vi "Framework.Create.Transfers.vi"(5 "Group String Buffer":refnum<class "Buffer.lvclass">, 7 "Group Intermediate Buffer":refnum<class "DBL Pointer.lvclass">, 8 "error in (no error)":errorcluster, 10 "Transfer Configurations":refnum<class "Transfer Configuration.lvclass">[](array[class]), 11 "Framework in":refnum<class "Framework.lvclass">) -> (0 "error out":errorcluster, 2 "Transfers":refnum<class "Transfer.lvclass">[](array[class]), 3 "Framework out":refnum<class "Framework.lvclass">)   [LabVIEW 2017, in "DSF Core.lvlib" / "Framework.lvclass"]
uses:
  Framework.lvclass
  Transfer/Transfer.lvclass
  Shared/Classes/Transfer/Transfer Configuration.lvclass
  Buffer/Buffer.lvclass
  C:/Program Files (x86)/National Instruments/LabVIEW 2017/vi.lib/NI/Memory Manager/Classes/Pointer/Memory.Pointer.lvclass
  Pointer/DBL Pointer.lvclass
  Framework.lvclass/Framework.ctl
  Cache/Cache.lvclass/Cache.ctl
  DSF Configuration API/Public/Controls/DSF Data Type.ctl
  <vilib>/NI/Memory Manager/Classes/Pointer/Memory.Pointer.lvclass/Memory.Pointer.ctl
  Shared/Classes/Transfer/Transfer Configuration.lvclass/Transfer Configuration.ctl
  Shared/VIs/Data Type.Sizeof.vi
  <vilib>/NI/Memory Manager/Classes/Pointer/Memory.Pointer.Parameter Check.Subset.vi
  <vilib>/NI/Memory Manager/Classes/Pointer/Memory.Pointer.Get Address.vi
  <vilib>/NI/Memory Manager/Classes/Pointer/Memory.Pointer.Encapsulate.vi
  <vilib>/NI/Memory Manager/Classes/Pointer/Memory.Pointer.Parameter Check.Null Pointer.vi
  <vilib>/NI/Memory Manager/Classes/Pointer/Memory.Pointer.Errors.vi
  <vilib>/NI/Memory Manager/Classes/Pointer/Memory.Pointer.Errors.Out of Bounds.vi
  <vilib>/NI/Memory Manager/Classes/Pointer/Memory.Pointer.Get Size.vi
  <vilib>/NI/Memory Manager/Classes/Pointer/Memory.Pointer.Set Size.vi
  <vilib>/NI/Memory Manager/Classes/Pointer/Memory.Pointer.Set Address.vi
  <vilib>/NI/Memory Manager/Classes/Pointer/Memory.Pointer.Set Allocated.vi
  <vilib>/NI/Memory Manager/Classes/Pointer/Memory.Pointer.Errors.Null Pointer.vi
  <vilib>/NI/Memory Manager/VIs/Source.Write.String.vi
  <vilib>/NI/Memory Manager/Classes/Pointer/Memory.Pointer.Errors.Write Pointer Size.vi
  <vilib>/NI/Memory Manager/Classes/Pointer/Memory.Pointer.Errors.Create Error.vi
  <vilib>/NI/Memory Manager/VIs/Source.Write.Scalar.Base10.vi
  <vilib>/NI/Memory Manager/VIs/Source.Write.Scalar.Base10 (U64).vi
  <vilib>/NI/Memory Manager/VIs/New Error Cluster Constant.vi
  <vilib>/NI/Memory Manager/VIs/New Error Cluster Constant (512B).vi
  <vilib>/NI/Memory Manager/VIs/Error Cluster.Set Status.vi
  <vilib>/NI/Memory Manager/VIs/Error Cluster.Set Code.vi
  <vilib>/NI/Memory Manager/VIs/Error Cluster.Set VI Source.vi
  <vilib>/NI/Memory Manager/Constants/Memory.Constants.vi
  <vilib>/NI/Memory Manager/Constants/Memory.Constants.Library Name.vi
  <vilib>/NI/Memory Manager/Classes/Pointer/Memory.Pointer.Errors.Get Info.vi
  Cache/Cache.lvclass
  DSF Core.lvlib
  <vilib>/NI/Memory Manager/Classes/Pointer/Memory.Pointer.lvclass
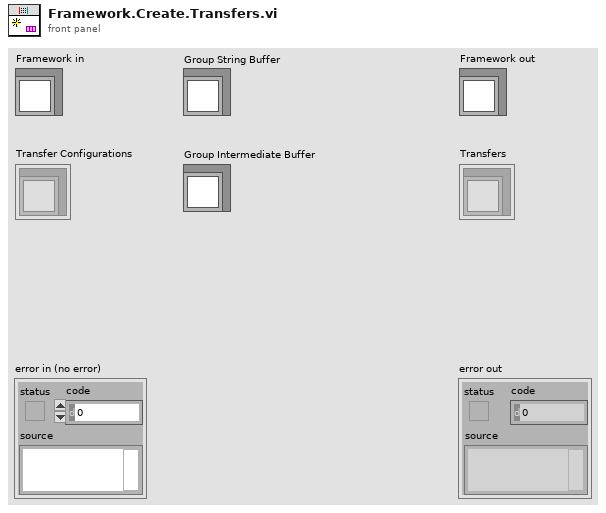
[diagram p1: front panel]
types:
  T1 = typedef "DSF Core.lvlib/DSF Data Type.ctl" = enum8{"Bool", "SGL", "DBL", "I8", "I16", "I32", "I64", "U8", "U16", "U32", "U64"}
  T2 = typedef "DSF Core.lvlib/DSF Runtime Channel Block.ctl" = cluster{"data type":T1, "count":u64, "buffer offset":u64}
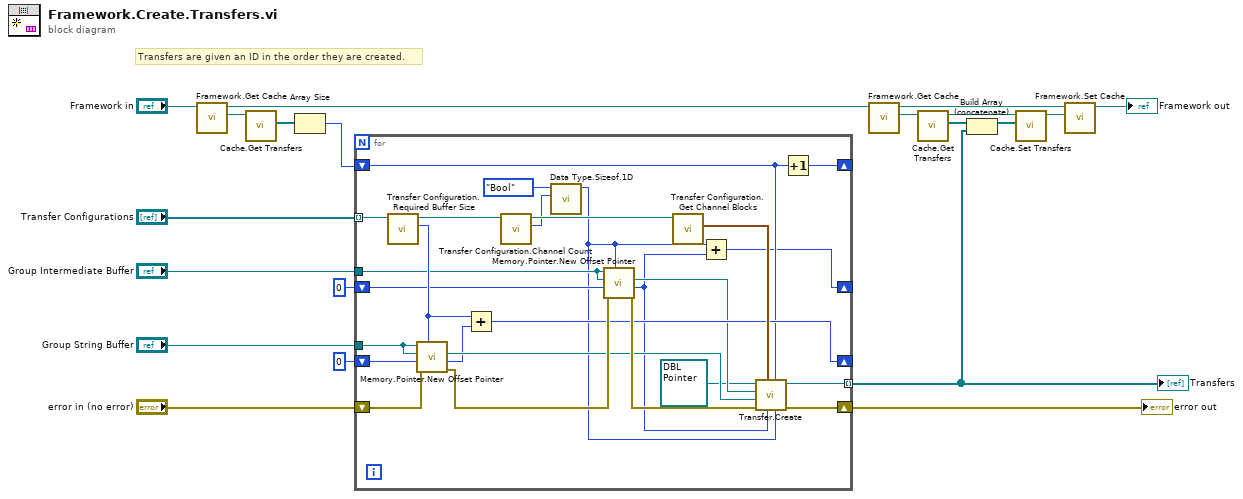
[diagram p0: block diagram]
diagram:
  # "Transfers are given an ID in the order they are created."
  n1 = call "Framework.Get Cache.vi"("Framework in"="Framework in") -> ("Cache"=w14:refnum<class "Cache.lvclass">, "Framework out"=w12:refnum<class "Framework.lvclass">)  [unwired: 9 in]
  n2 = call "Cache.Get Transfers.vi"("Cache in"=w14) -> ("Transfers"=w16:refnum<class "Transfer.lvclass">[])  [unwired: 9 in, 1 out]
  n3 = Array Size(array=w16) -> (size(s)=w17:i32)
  n4 = for {
    shift-right: [w44] -> w20
    shift-left: "error in (no error)" -> [w33]
    tunnel: [w43] -> w10 mode=indexing
    tunnel: "Transfer Configurations" -> [w41] mode=indexing
    tunnel: "Group Intermediate Buffer" -> [w26]
    shift-right: [w27] -> _
    shift-left: u64 0 -> [w24]
    tunnel: "Group String Buffer" -> [w31]
    shift-right: [w35] -> _
    shift-left: u64 0 -> [w39]
    shift-right: [w29] -> _
    shift-left: w17 -> [w28]
    n5 = call "Transfer Configuration.Required Buffer Size.vi"("Transfer Configuration in"=w41) -> ("required buffer size"=w38:u64, "Transfer Configuration out"=w40:refnum<class "Transfer Configuration.lvclass">)  [unwired: 8 in, 1 out]
    n6 = call <vilib>:"Memory.Pointer.New Offset Pointer.vi"("length (-1: rest)"=w38, "error in (no error)"=w33, "offset (0)"=w39, "offset Pointer type"=w31, "base Pointer in"=w31) -> ("error out"=w46:errorcluster, "offset out"=w32:u64, "offset Pointer"=w37:refnum<class "Buffer.lvclass">)  [unwired: 3 in, 1 out]
    n7 = Add(x=w38, y=w32) -> (x+y=w35:u64)
    n8 = call "Transfer Configuration.Channel Count.vi"("Transfer Configuration in"=w40) -> ("total channel count"=w30:u64, "Transfer Configuration out"=w34:refnum<class "Transfer Configuration.lvclass">)  [unwired: 8 in, 1 out]
    n9 = call "Data Type.Sizeof.1D.vi"("count"=w30, "data type"=DSF_Data_Type."Bool") -> ("size in bytes"=w21:u64)  [unwired: 9 in]
    n10 = call <vilib>:"Memory.Pointer.New Offset Pointer.vi"("length (-1: rest)"=w21, "error in (no error)"=w46, "offset (0)"=w24, "offset Pointer type"=w26, "base Pointer in"=w26) -> ("error out"=w45:errorcluster, "offset out"=w22:u64, "offset Pointer"=w25:refnum<class "DBL Pointer.lvclass">)  [unwired: 3 in, 1 out]
    n11 = call "Transfer Configuration.Get Channel Blocks.vi"("Transfer Configuration in"=w34) -> ("channel blocks"=w36:T2[])  [unwired: 9 in, 1 out]
    n12 = Add(x=w21, y=w22) -> (x+y=w27:u64)
    n13 = call "Transfer.Create.vi"("size"=w21, "id"=w28, "group offset"=w22, "channel blocks"=w36, "error in (no error)"=w45, "String Buffer"=w37, "Intermediate Buffer"=w25, "Inline Buffer"=refnum<class "DBL Pointer.lvclass"> refnum) -> ("error out"=w44:errorcluster, "Transfer out"=w43:refnum<class "Transfer.lvclass">)  [unwired: 2 in]
    n14 = Increment(x=w28) -> (x+1=w29:i32)
  }
  "error out" <- w20
  "Transfers" <- w10
  n15 = call "Framework.Get Cache.vi"("Framework in"=w12) -> ("Cache"=w13:refnum<class "Cache.lvclass">, "Framework out"=w9:refnum<class "Framework.lvclass">)  [unwired: 9 in]
  n16 = call "Cache.Get Transfers.vi"("Cache in"=w13) -> ("Transfers"=w11:refnum<class "Transfer.lvclass">[], "Cache out"=w5:refnum<class "Cache.lvclass">)  [unwired: 9 in]
  n17 = Build Array (concatenate)(w11, w10) -> (w8:refnum<class "Transfer.lvclass">[])
  n18 = call "Cache.Set Transfers.vi"("Transfers"=w8, "Cache in"=w5) -> ("Cache out"=w7:refnum<class "Cache.lvclass">)  [unwired: 9 in]
  n19 = call "Framework.Set Cache.vi"("Cache"=w7, "Framework in"=w9) -> ("Framework out"=→"Framework out":refnum<class "Framework.lvclass">)  [unwired: 9 in]
